vi "Write Display.vi"(8 "error in (no error)":errorcluster, 9 "Display On":bool, 10 "Session In":refnum<class "Session.lvclass">, 11 "PCF8574 I2C LCD I in":refnum<class "PCF8574 I2C LCD.lvclass">) -> (0 "error out":errorcluster, 2 "Session Out":refnum<class "Session.lvclass">, 3 "PCF8574 I2C LCD I out":refnum<class "PCF8574 I2C LCD.lvclass">)   [LabVIEW 2020, in "CTI-Peripheral.lvlib" / "PCF8574 I2C LCD.lvclass"]
uses:
  PCF8574 I2C LCD.lvclass
  CTI/Session/Session.lvclass
  PCF8574 I2C LCD.lvclass/PCF8574 I2C LCD.ctl
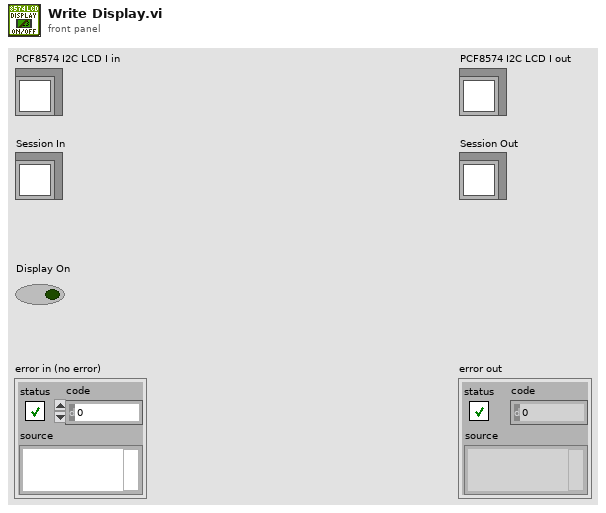
[diagram p1: front panel]
types:
  T1 = typedef "CTI-Peripheral.lvlib/HD44780 LCD.lvlib/Display Control.ctl" = cluster{"Blink On":bool, "Cursor On":bool, "Display On":bool}
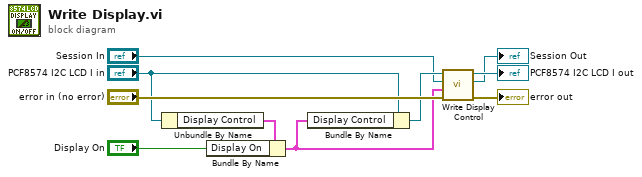
[diagram p0: block diagram]
diagram:
  n1 = Unbundle By Name("PCF8574 I2C LCD I in") -> ("Display Control"=w8:T1)
  n2 = Bundle By Name(cluster=w8, "Display On"="Display On") -> (w3:T1)
  n3 = Bundle By Name(cluster="PCF8574 I2C LCD I in", "Display Control"=w3) -> (w5:refnum<class "PCF8574 I2C LCD.lvclass">)
  n4 = call "Write Display Control.vi"("error in (no error)"="error in (no error)", "Display Control"=w3, "Session In"="Session In", "PCF8574 I2C LCD in"=w5) -> ("error out"=→"error out":errorcluster, "Session Out"=→"Session Out":refnum<class "Session.lvclass">, "PCF8574 I2C LCD out"=→"PCF8574 I2C LCD I out":refnum<class "PCF8574 I2C LCD.lvclass">)  [unwired: 5 in]
